vi "Sep_Flow_Control.vi"(11 "kill process":bool) -> ()   [LabVIEW 2019]
uses:
  <vilib>/Utility/config.llb/Read Key (String).vi
  <vilib>/Instr/_visa.llb/VISA Configure Serial Port (Instr).vi
  <vilib>/Utility/config.llb/Read Key (Path).vi
  <vilib>/Utility/file.llb/Read From Spreadsheet File (DBL).vi
  <vilib>/Utility/config.llb/NI_LVConfig.lvlib
panel:
  in  "Scale Selectors":enum32{"0-100 SLM", "0-10 SLM", "0-1 SLM"}(radio)
  out "concatenated string":string
  in  "Enter the Set Point for the Flow":string
  in  "Please Close the Program After \nSetting the Flow":bool
  out "Acknowledgement":string
  out "Separator Flow":cluster{dbl[], dbl[]}(graph)
  in  "close":bool
  in  "open":bool
  out "error out 2":errorcluster
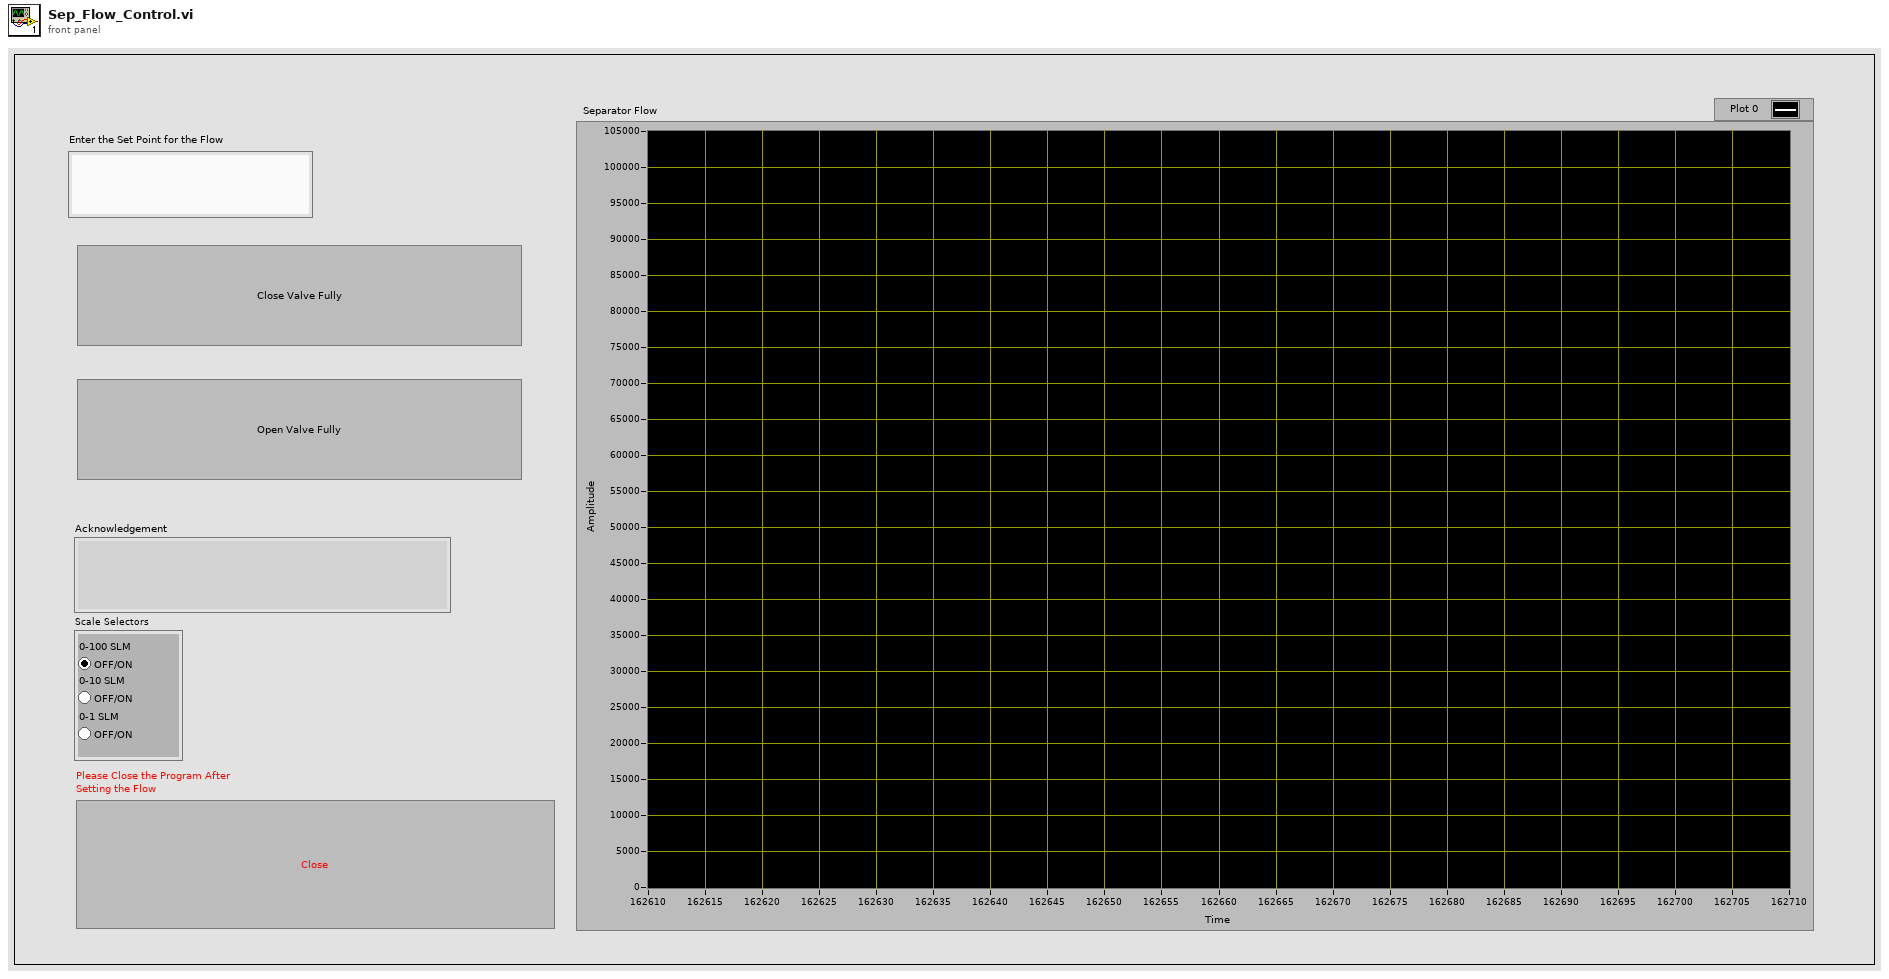
[diagram p1: front panel]
types:
  T1 = typedef "NI_LVConfig.lvlib/Config Data RefNum.ctl" = refnum<k1>
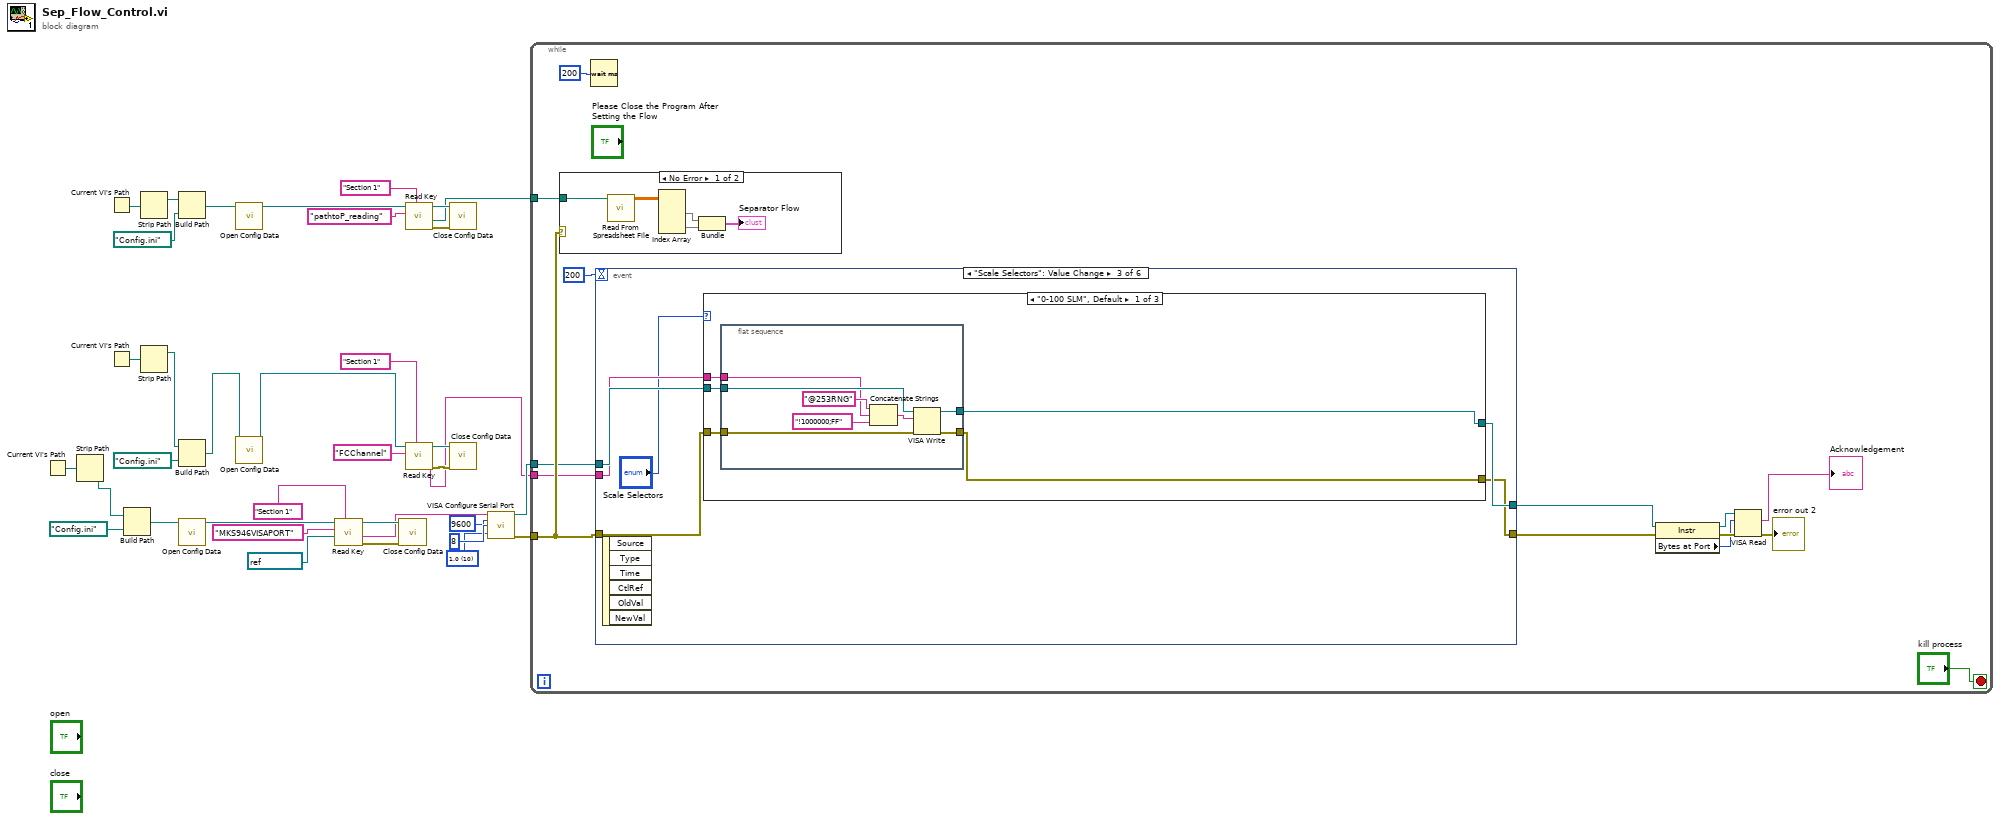
[diagram p0: block diagram]
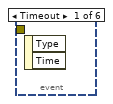
[diagram p2: hidden frame]
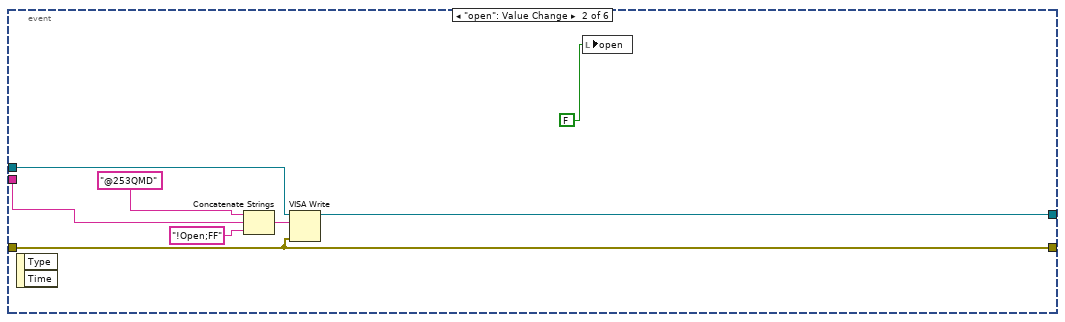
[diagram p3: hidden frame]
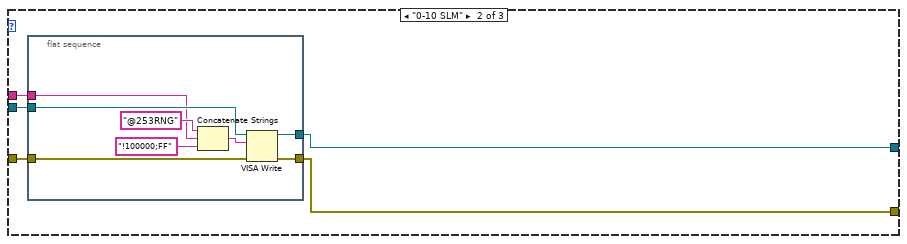
[diagram p4: hidden frame]
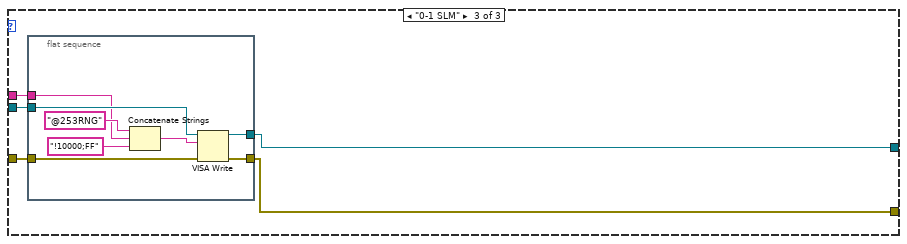
[diagram p5: hidden frame]
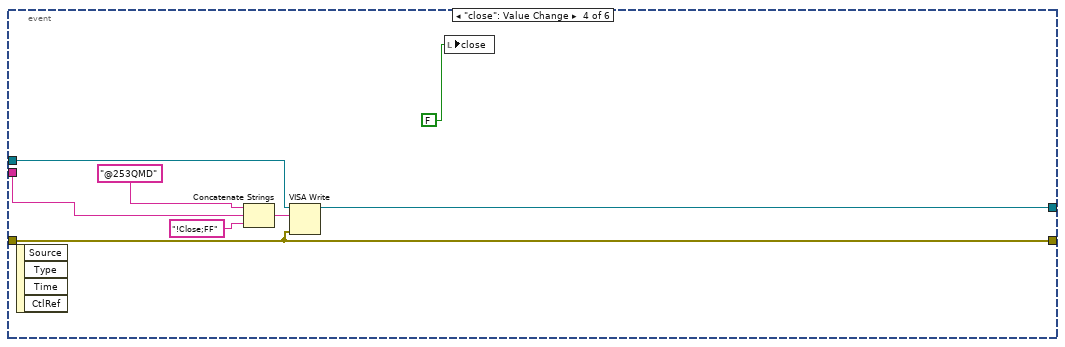
[diagram p6: hidden frame]
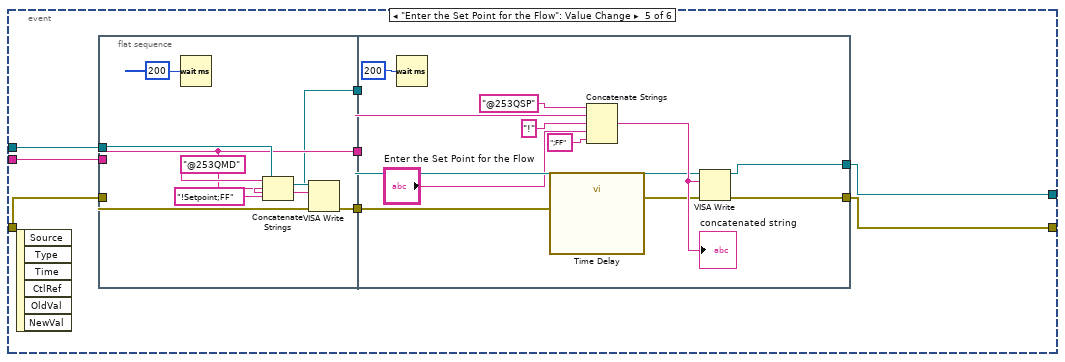
[diagram p7: hidden frame]
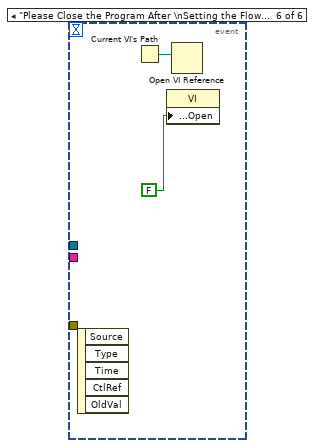
[diagram p8: hidden frame]
diagram:
  w34 = u16 10 items=["1.0"=10, "1.5"=15, "2.0"=20] ("stop bits (10: 1 bit)")
  n1 = Current VI's Path() -> (path=w4:path)
  n2 = Strip Path(path=w4) -> (stripped path=w3:path)  [unwired: 1 out]
  n3 = Current VI's Path() -> (path=w2:path)
  n4 = Current VI's Path() -> (path=w6:path)
  n5 = Build Path(base path=w3, name or relative path=path "Config.ini" ("default name")) -> (appended path=w28:path)
  n6 = Strip Path(path=w2) -> (stripped path=w1:path)  [unwired: 1 out]
  n7 = Strip Path(path=w6) -> (stripped path=w5:path)  [unwired: 1 out]
  n8 = Build Path(base path=w1, name or relative path=path "Config.ini" ("default name")) -> (appended path=w19:path)
  n9 = Build Path(base path=w5, name or relative path=path "Config.ini" ("default name")) -> (appended path=w9:path)
  n10 = call <vilib>:"Open Config Data.vi"("configuration file path"=w28) -> ("refnum"=w33:T1)  [unwired: 8 in, 2 out]
  n11 = call <vilib>:"Open Config Data.vi"("configuration file path"=w19) -> ("refnum"=w24:T1)  [unwired: 8 in, 2 out]
  n12 = call <vilib>:"Open Config Data.vi"("configuration file path"=w9) -> ("refnum"=w14:T1)  [unwired: 8 in, 2 out]
  n13 = call-poly <vilib>:"Read Key.vi"("section"="Section 1", "default value"=refnum<visa-resource-name> "COM5" ("VISA resource name"), "key"="MKS946VISAPORT", "refnum"=w33) -> ("error out"=w27:errorcluster, "value"=w25:string, "refnum out"=w31:T1)  [unwired: 4 in, 1 out]
  n14 = call <vilib>:"Close Config Data.vi"("error in (no error)"=w27, "refnum"=w31) -> ()  [unwired: 8 in, 2 out]
  n15 = call-poly <vilib>:"Read Key.vi"("section"="Section 1", "key"="pathtoP_reading", "refnum"=w24) -> ("error out"=w18:errorcluster, "value"=w17:path, "refnum out"=w22:T1)  [unwired: 5 in, 1 out]
  n16 = call-poly <vilib>:"Read Key.vi"("section"="Section 1", "key"="FCChannel", "refnum"=w14) -> ("error out"=w8:errorcluster, "value"=w7:string, "refnum out"=w12:T1)  [unwired: 5 in, 1 out]
  n17 = call <vilib>:"Close Config Data.vi"("error in (no error)"=w18, "refnum"=w22) -> ()  [unwired: 8 in, 2 out]
  n18 = call <vilib>:"Close Config Data.vi"("error in (no error)"=w8, "refnum"=w12) -> ()  [unwired: 8 in, 2 out]
  n19 = call-poly "VISA Configure Serial Port"("VISA resource name"=w25, "baud rate (9600)"=u32 9600, "data bits (8)"=u16 8, "stop bits (10: 1 bit)"=w34) -> ("VISA resource name out"=w15:refnum<visa-resource-name>, "error out"=w16:errorcluster)  [unwired: 10 in]
  n20 = while {
    tunnel: w17 -> [w50]
    tunnel: w16 -> [w46]
    tunnel: w15 -> [w42]
    tunnel: w7 -> [w43]
    stop <- "kill process" stop-if-true
    n21 = case shown="No Error" w46 {
      tunnel: w50 -> [w147 _]
      frame No Error {
        n22 = call-poly <vilib>:"Read From Spreadsheet File.vi"("file path (dialog if empty)"=w147) -> ("all rows"=w143:dbl[][])  [unwired: 6 in, 4 out]
        n23 = Index Array(array=w143) -> (element #1=w146:dbl[], element #2=w145:dbl[])  [unwired: 4 in]
        n24 = Bundle("all rows"=w146, "all rows"=w145) -> (→"Separator Flow":cluster{"all rows":dbl[], "all rows":dbl[]})  [unwired: 1 in]
      }
      frame Error {
      }
    }
    n25 = Wait (ms)(milliseconds to wait=u32 200) -> ()  [unwired: 1 out]
    n26 = event shown="[2] \"Scale Selectors\": Value Change" {
      selector: _ -> [_ _ _ _ _ _]
      dyn-events: _ -> [_ _ _ _ _ _]
      timeout: 200 -> [_ _ _ _ _ _]
      tunnel: w46 -> [_ w55 w63 w108 w119 _]
      tunnel: [_ w55 w59 w108 w115 _] -> w40
      tunnel: w42 -> [_ w52 w64 w105 w118 _]
      tunnel: w43 -> [_ w56 w62 w109 w117 _]
      tunnel: [_ w53 w60 w106 w112 _] -> w41
      event Timeout {
        n27 = event-data() -> ()  [unwired: 1 in, 2 out]
      }
      event "open": Value Change {
        n28 = event-data() -> ()  [unwired: 1 in, 2 out]
        n29 = Concatenate Strings("@253QMD", w56, "!Open;FF") -> (w54:string)
        n30 = VISA Write(VISA resource name=w52, write buffer=w54, error in (no error)=w55) -> (VISA resource name out=w53:refnum<visa-resource-name>)  [unwired: 2 out]
        n31 = local write "open"(FALSE ("open")) -> ()
      }
      event "Scale Selectors": Value Change {
        n32 = event-data() -> ()  [unwired: 1 in, 6 out]
        n33 = case shown="\"0-100 SLM\", Default" "Scale Selectors" {
          tunnel: w64 -> [w68 w81 w93]
          tunnel: w63 -> [w67 w80 w94]
          tunnel: w62 -> [w69 w82 w95]
          tunnel: [w65 w79 w92] -> w60
          tunnel: [w66 w78 w91] -> w59
          frame "0-100 SLM", Default {
            n34 = flat-sequence {
              tunnel: w69 -> [w72]
              tunnel: w67 -> [w74]
              tunnel: w68 -> [w73]
              tunnel: [w71] -> w65
              tunnel: [w70] -> w66
              frame #0 {
                n35 = Concatenate Strings("@253RNG", w72, "!1000000;FF") -> (w75:string)
                n36 = VISA Write(VISA resource name=w73, write buffer=w75, error in (no error)=w74) -> (VISA resource name out=w71:refnum<visa-resource-name>, error out=w70:errorcluster)  [unwired: 1 out]
              }
            }
          }
          frame "0-10 SLM" {
            n37 = flat-sequence {
              tunnel: w82 -> [w85]
              tunnel: w80 -> [w87]
              tunnel: w81 -> [w86]
              tunnel: [w84] -> w79
              tunnel: [w83] -> w78
              frame #0 {
                n38 = Concatenate Strings("@253RNG", w85, "!100000;FF") -> (w88:string)
                n39 = VISA Write(VISA resource name=w86, write buffer=w88, error in (no error)=w87) -> (VISA resource name out=w84:refnum<visa-resource-name>, error out=w83:errorcluster)  [unwired: 1 out]
              }
            }
          }
          frame "0-1 SLM" {
            n40 = flat-sequence {
              tunnel: w95 -> [w98]
              tunnel: w94 -> [w100]
              tunnel: w93 -> [w99]
              tunnel: [w97] -> w92
              tunnel: [w96] -> w91
              frame #0 {
                n41 = Concatenate Strings("@253RNG", w98, "!10000;FF") -> (w101:string)
                n42 = VISA Write(VISA resource name=w99, write buffer=w101, error in (no error)=w100) -> (VISA resource name out=w97:refnum<visa-resource-name>, error out=w96:errorcluster)  [unwired: 1 out]
              }
            }
          }
        }
      }
      event "close": Value Change {
        n43 = event-data() -> ()  [unwired: 1 in, 4 out]
        n44 = Concatenate Strings("@253QMD", w109, "!Close;FF") -> (w107:string)
        n45 = VISA Write(VISA resource name=w105, write buffer=w107, error in (no error)=w108) -> (VISA resource name out=w106:refnum<visa-resource-name>)  [unwired: 2 out]
        n46 = local write "close"(FALSE ("close")) -> ()
      }
      event "Enter the Set Point for the Flow": Value Change {
        n47 = event-data() -> ()  [unwired: 1 in, 6 out]
        n48 = flat-sequence {
          tunnel: w119 -> [w127]
          tunnel: w118 -> [w126]
          tunnel: w117 -> [w122]
          tunnel: [w122] -> w116
          tunnel: [w121] -> w114
          tunnel: [w120] -> w113
          tunnel: w116 -> [w139]
          tunnel: [w134] -> w115
          tunnel: w114 -> [w133]
          tunnel: w113 -> [w132]
          tunnel: [w129] -> w112
          frame #0 {
            n49 = Wait (ms)(milliseconds to wait=u32 200) -> ()  [unwired: 1 out]
            n50 = Concatenate Strings("@253QMD", w122, "!Setpoint;FF") -> (w124:string)
            n51 = VISA Write(VISA resource name=w126, write buffer=w124, error in (no error)=w127) -> (VISA resource name out=w121:refnum<visa-resource-name>, error out=w120:errorcluster)  [unwired: 1 out]
          }
          frame #1 {
            n52 = Wait (ms)(milliseconds to wait=u32 200) -> ()  [unwired: 1 out]
            n53 = call "Time Delay"("error in (no error)"=w132) -> ("error out"=w131:errorcluster)  [unwired: 10 in]
            n54 = Concatenate Strings("@253QSP", w139, "!", "Enter the Set Point for the Flow", ";FF") -> (w135:string)
            "concatenated string" <- w135
            n55 = VISA Write(VISA resource name=w133, write buffer=w135, error in (no error)=w131) -> (VISA resource name out=w129:refnum<visa-resource-name>, error out=w134:errorcluster)  [unwired: 1 out]
          }
        }
      }
      event "Please Close the Program After \nSetting the Flow": Value Change {
        n56 = event-data() -> ()  [unwired: 1 in, 5 out]
        n57 = Current VI's Path() -> (path=w141:path)
        n58 = property class="VI"("Front Panel Window:Open"=FALSE) -> ()  [unwired: 2 in, 2 out]
        n59 = Open VI Reference(vi path=w141) -> ()  [unwired: 5 in, 2 out]
      }
    }
    n60 = property class="Instr"(reference=w41, error in=w40) -> (reference out=w47:refnum<visa-resource-name>, error out=w49:errorcluster, "Bytes at Port"=w48:u32)
    n61 = VISA Read(VISA resource name=w47, byte count=w48, error in (no error)=w49) -> (read buffer=→"Acknowledgement":string, error out=→"error out 2":errorcluster)  [unwired: 2 out]
  }
